vi "TDC_enableHbt.vi"(8 "Error In":errorcluster, 9 "Enable":bool=TRUE) -> (0 "Error Out":errorcluster)   [LabVIEW 2011]
uses:
  tdcbase.dll
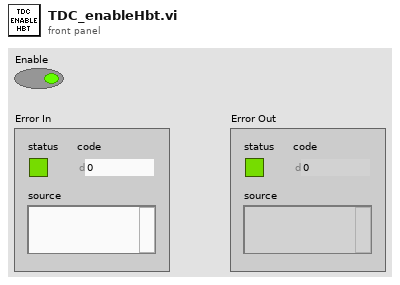
[diagram p1: front panel]
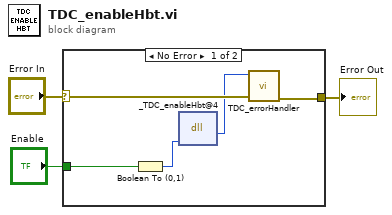
[diagram p0: block diagram]
diagram:
  n1 = case shown="No Error" "Error In" {
    selector: "Error In" -> [w7 w9]
    tunnel: [w6 w9] -> w2
    tunnel: "Enable" -> [w4 _]
    frame No Error {
      n2 = Boolean To (0,1)(Boolean=w4) -> (0, 1=w8:i16)
      n3 = dll-call lib="X:/tdcbase.dll" fn="_TDC_enableHbt@4"("enable"=w8) -> ("return type"=w5:i32)  [unwired: 4 in, 2 out]
      n4 = call "TDC_errorHandler.vi"("Error In"=w7, "TDC Return Code"=w5) -> ("Error Out"=w6:errorcluster)  [unwired: 9 in]
    }
    frame Error {
    }
  }
  "Error Out" <- w2
